vi "Obtain Broadcast Events.vi"(8 "error in (no error)":errorcluster, 10 "Create New? (F)":bool) -> (0 "error out":errorcluster, 2 "NI DAQ Broadcast Events":T1)   [LabVIEW 2020, in "NI DAQ.lvlib"]
doc: "This VI Obtains/Creates the Broadcast events that will be used for other modules to register to receive messages from the module that owns this VI.\n\n<b>NOTE</b>: The contents of this VI are automatically generated and modified by the <b>Tools > Delacor > DQMH</b> utilities. Consider using those utilities instead of making your own modifications to this VI.\n_____\nBased on DQMH Project Template 6.1.0.94."
uses:
  NI DAQ.lvlib
  Broadcast Events--cluster.ctl
  Did Init Argument--cluster.ctl
  Status Updated Argument--cluster.ctl
  Error Reported Argument--cluster.ctl
  Stop Argument--cluster.ctl
  Get Module Execution Status Argument--cluster.ctl
  Digital data acquired Argument--cluster.ctl
  Device connected Argument--cluster.ctl
  Connection failed Argument--cluster.ctl
  Analog data acquired Argument--cluster.ctl
  Counter data acquired Argument--cluster.ctl
  Temperature data acquired Argument--cluster.ctl
panel:
  # "NOTE: The contents of this VI are automatically generated and modified by the Tools > Delacor > DQMH utilities. Consider using those utilities instead of making your own modifications to this VI."
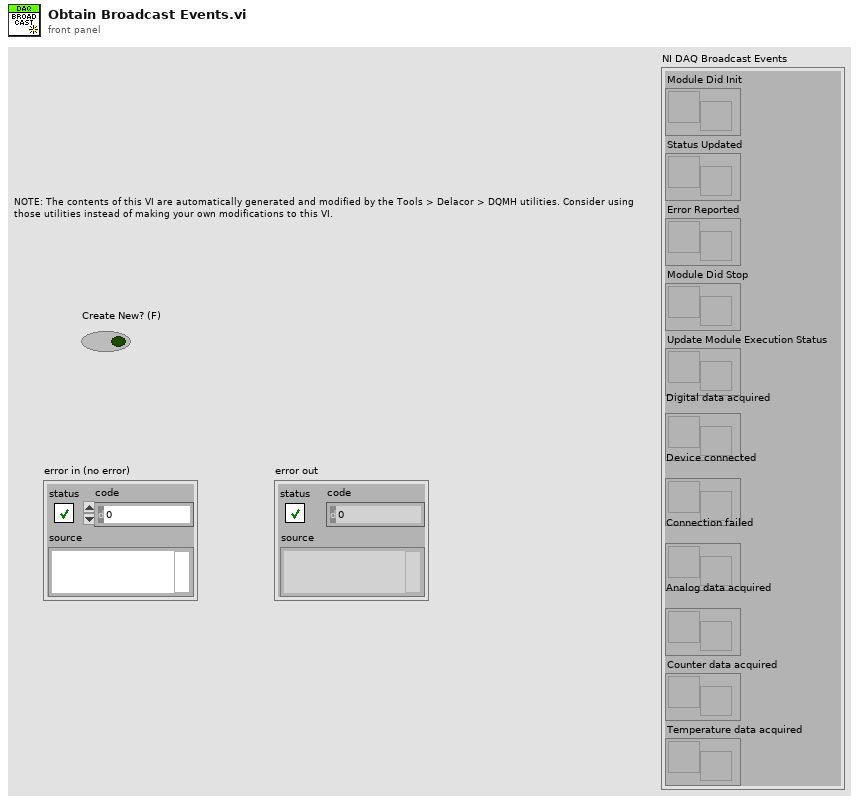
[diagram p1: front panel]
types:
  T1 = typedef "NI DAQ.lvlib/Broadcast Events--cluster.ctl" = cluster{"Module Did Init":refnum<user-event>, "Status Updated":refnum<user-event>, "Error Reported":refnum<user-event>, "Module Did Stop":refnum<user-event>, "Update Module Execution Status":refnum<user-event>, "Digital data acquired":refnum<user-event>, "Device connected":refnum<user-event>, "Connection failed":refnum<user-event>, "Analog data acquired":refnum<user-event>, "Counter data acquired":refnum<user-event>, "Temperature data acquired":refnum<user-event>}
  T2 = typedef "NI DAQ.lvlib/Temperature data acquired Argument--cluster.ctl" = cluster{"Module ID":i32, "Temperature":dbl}
  T3 = typedef "NI DAQ.lvlib/Counter data acquired Argument--cluster.ctl" = cluster{"Module ID":i32, "Data":dbl[]}
  T4 = typedef "NI DAQ.lvlib/Analog data acquired Argument--cluster.ctl" = cluster{"Module ID":i32, "Data":dbl[]}
  T5 = typedef "NI DAQ.lvlib/Connection failed Argument--cluster.ctl" = cluster{"Module ID":i32, "Connected?":bool}
  T6 = typedef "NI DAQ.lvlib/Device connected Argument--cluster.ctl" = cluster{"Module ID":i32, "Connected?":bool}
  T7 = typedef "NI DAQ.lvlib/Digital data acquired Argument--cluster.ctl" = cluster{"Module ID":i32, "Data":bool[]}
  T8 = typedef "NI DAQ.lvlib/Get Module Execution Status Argument--cluster.ctl" = cluster{"Module ID":i32, "Running?":bool}
  T9 = typedef "NI DAQ.lvlib/Stop Argument--cluster.ctl" = cluster{"Module ID":i32, "Origin":string, "Exit via Stop Module Req?":bool, "Wait for Module to stop?":bool}
  T10 = typedef "NI DAQ.lvlib/Error Reported Argument--cluster.ctl" = cluster{"Error":errorcluster, "Additional Information":string, "Module ID":i32, "Module Name":string}
  T11 = typedef "NI DAQ.lvlib/Status Updated Argument--cluster.ctl" = cluster{"Status":string, "Module ID":i32}
  T12 = typedef "NI DAQ.lvlib/Did Init Argument--cluster.ctl" = cluster{"Init?":bool, "Info":string, "Module ID":i32}
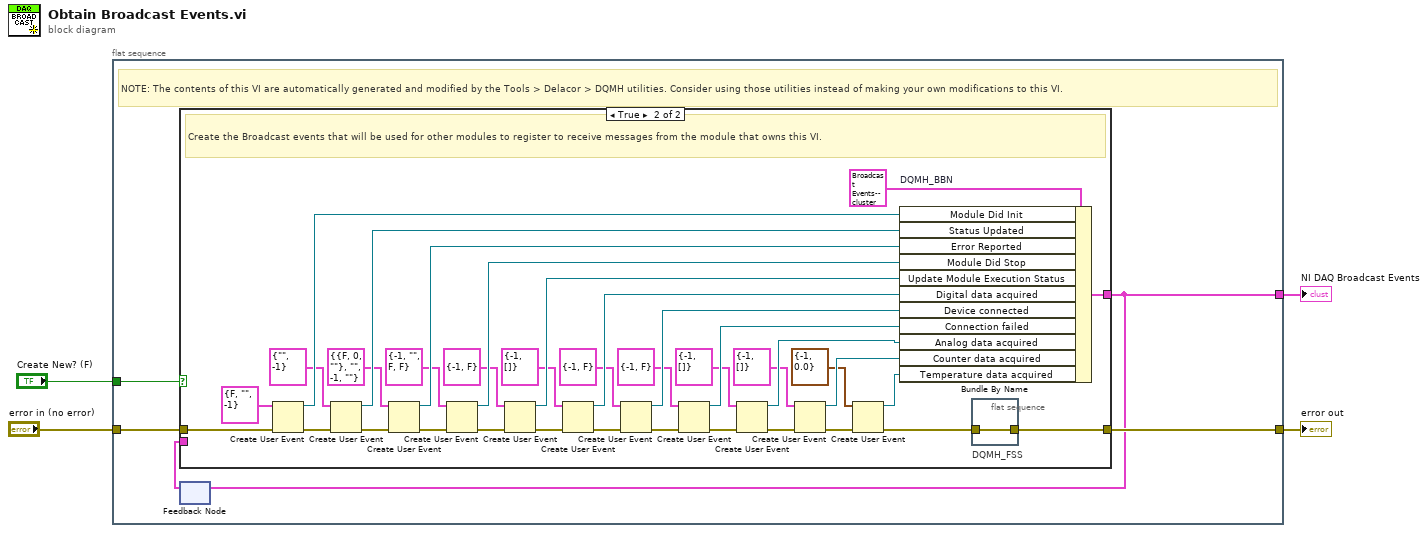
[diagram p0: block diagram]
diagram:
  n1 = flat-sequence {
    tunnel: [w9] -> w4
    tunnel: "error in (no error)" -> [w8]
    tunnel: [w6] -> w2
    tunnel: "Create New? (F)" -> [w5]
    frame #0 {
      # "NOTE: The contents of this VI are automatically generated and modified by the Tools > Delacor > DQMH utilities. Consider using those utilities instead of making your own modifications to this VI."
      n2 = feedback #1() -> (w7:T1)  [unwired: 1 in]
      n3 = case shown="True" w5 {
        tunnel: [w10 w33] -> w9
        tunnel: w8 -> [w10 w48]
        tunnel: [w11 w45] -> w6
        tunnel: w7 -> [w11 _]
        frame False {
          # "Obtain the Broadcast events that were created in a previous call to this VI."
        }
        frame True {
          # "Create the Broadcast events that will be used for other modules to register to receive messages from the module that owns this VI."
          n4 = Create User Event(user event datatype=T12 {"Init?"=FALSE, "Info"="", "Module ID"=-1} ("Did Init Argument"), error in=w48) -> (user event=w46:refnum<user-event>, error out=w43:errorcluster)
          n5 = Create User Event(user event datatype=T11 {"Status"="", "Module ID"=-1} ("Status Updated Argument"), error in=w43) -> (user event=w40:refnum<user-event>, error out=w42:errorcluster)
          n6 = Create User Event(user event datatype=T10 {"Error"={"status"=FALSE, "code"=0, "source"=""}, "Additional Information"="", "Module ID"=-1, "Module Name"=""} ("Error Reported Argument"), error in=w42) -> (user event=w37:refnum<user-event>, error out=w39:errorcluster)
          n7 = Create User Event(user event datatype=T9 {"Module ID"=-1, "Origin"="", "Exit via Stop Module Req?"=FALSE, "Wait for Module to stop?"=FALSE} ("Stop Argument"), error in=w39) -> (user event=w35:refnum<user-event>, error out=w34:errorcluster)
          n8 = Create User Event(user event datatype=T8 {"Module ID"=-1, "Running?"=FALSE} ("Get Module Execution Status Argument"), error in=w34) -> (user event=w31:refnum<user-event>, error out=w32:errorcluster)
          n9 = Create User Event(user event datatype=T7 {"Module ID"=-1, "Data"=[]} ("Data acquired Argument"), error in=w32) -> (user event=w28:refnum<user-event>, error out=w29:errorcluster)
          n10 = Create User Event(user event datatype=T6 {"Module ID"=-1, "Connected?"=FALSE} ("Device connected Argument"), error in=w29) -> (user event=w25:refnum<user-event>, error out=w26:errorcluster)
          n11 = Create User Event(user event datatype=T5 {"Module ID"=-1, "Connected?"=FALSE} ("Connection failed Argument"), error in=w26) -> (user event=w22:refnum<user-event>, error out=w23:errorcluster)
          n12 = Create User Event(user event datatype=T4 {"Module ID"=-1, "Data"=[]} ("Analog data acquired Argument"), error in=w23) -> (user event=w19:refnum<user-event>, error out=w20:errorcluster)
          n13 = Create User Event(user event datatype=T3 {"Module ID"=-1, "Data"=[]} ("Counter data acquired Argument"), error in=w20) -> (user event=w16:refnum<user-event>, error out=w17:errorcluster)
          n14 = Create User Event(user event datatype=T2 {"Module ID"=-1, "Temperature"=0.0} ("Temperature data acquired Argument"), error in=w17) -> (user event=w13:refnum<user-event>, error out=w14:errorcluster)
          n15 = Bundle By Name "DQMH_BBN"(cluster=T1 {"Module Did Init"=refnum, "Status Updated"=refnum, "Error Reported"=refnum, "Module Did Stop"=refnum, "Update Module Execution Status"=refnum, "Digital data acquired"=refnum, "Device connected"=refnum, "Connection failed"=refnum, "Analog data acquired"=refnum, "Counter data acquired"=refnum, "Temperature data acquired"=refnum} ("output cluster"), "Module Did Init"=w46, "Status Updated"=w40, "Error Reported"=w37, "Module Did Stop"=w35, "Update Module Execution Status"=w31, "Digital data acquired"=w28, "Device connected"=w25, "Connection failed"=w22, "Analog data acquired"=w19, "Counter data acquired"=w16, "Temperature data acquired"=w13) -> (w45:T1)
          n16 = flat-sequence "DQMH_FSS" {
            tunnel: w14 -> [w49]
            tunnel: [w49] -> w33
            frame #0 {
            }
          }
        }
      }
      n17 = feedback-in #1(w6) -> ()
    }
  }
  "NI DAQ Broadcast Events" <- w2
  "error out" <- w4
